vi "Test MQTT-3.1.4-2.vi"(8 "error in (no error)":errorcluster) -> (0 "error out":errorcluster)   [LabVIEW 2013]
uses:
  <vilib>/LabVIEW Open Source Project/MQTT Control Packets/Control Packets/CONNACK/Connect Return Code -- enum.ctl
  <vilib>/LabVIEW Open Source Project/MQTT Control Packets/Control Packets/CONNACK/CONNACK.lvclass
  <vilib>/LabVIEW Open Source Project/MQTT Control Packets/Control Packets/CONNECT/CONNECT.lvclass
  <vilib>/LabVIEW Open Source Project/MQTT Control Packets/Control Packets/ControlPacket/ControlPacket.lvclass
  <vilib>/addons/_JKI Toolkits/Caraya/classes/Test/Test.lvclass
  <vilib>/addons/_JKI Toolkits/Caraya/classes/Assert/Assert.lvclass
  <vilib>/LabVIEW Open Source Project/MQTT Control Packets/Control Packets/DISCONNECT/DISCONNECT.lvclass
  <vilib>/LabVIEW Open Source Project/MQTT Connection/MQTT_Connection/Connection/Connection.lvclass
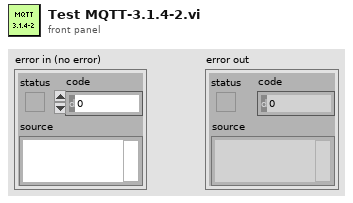
[diagram p1: front panel]
types:
  T1 = typedef "MQTT_Control_Packets.lvlib/CONNACK.lvclass/Connect Return Code -- enum.ctl" = enum16{"Connection accepted", "Unacceptable protocol version", "Identifier Rejected", "Server Unavailable", "Bad Username or Password", "Not Authorized"}
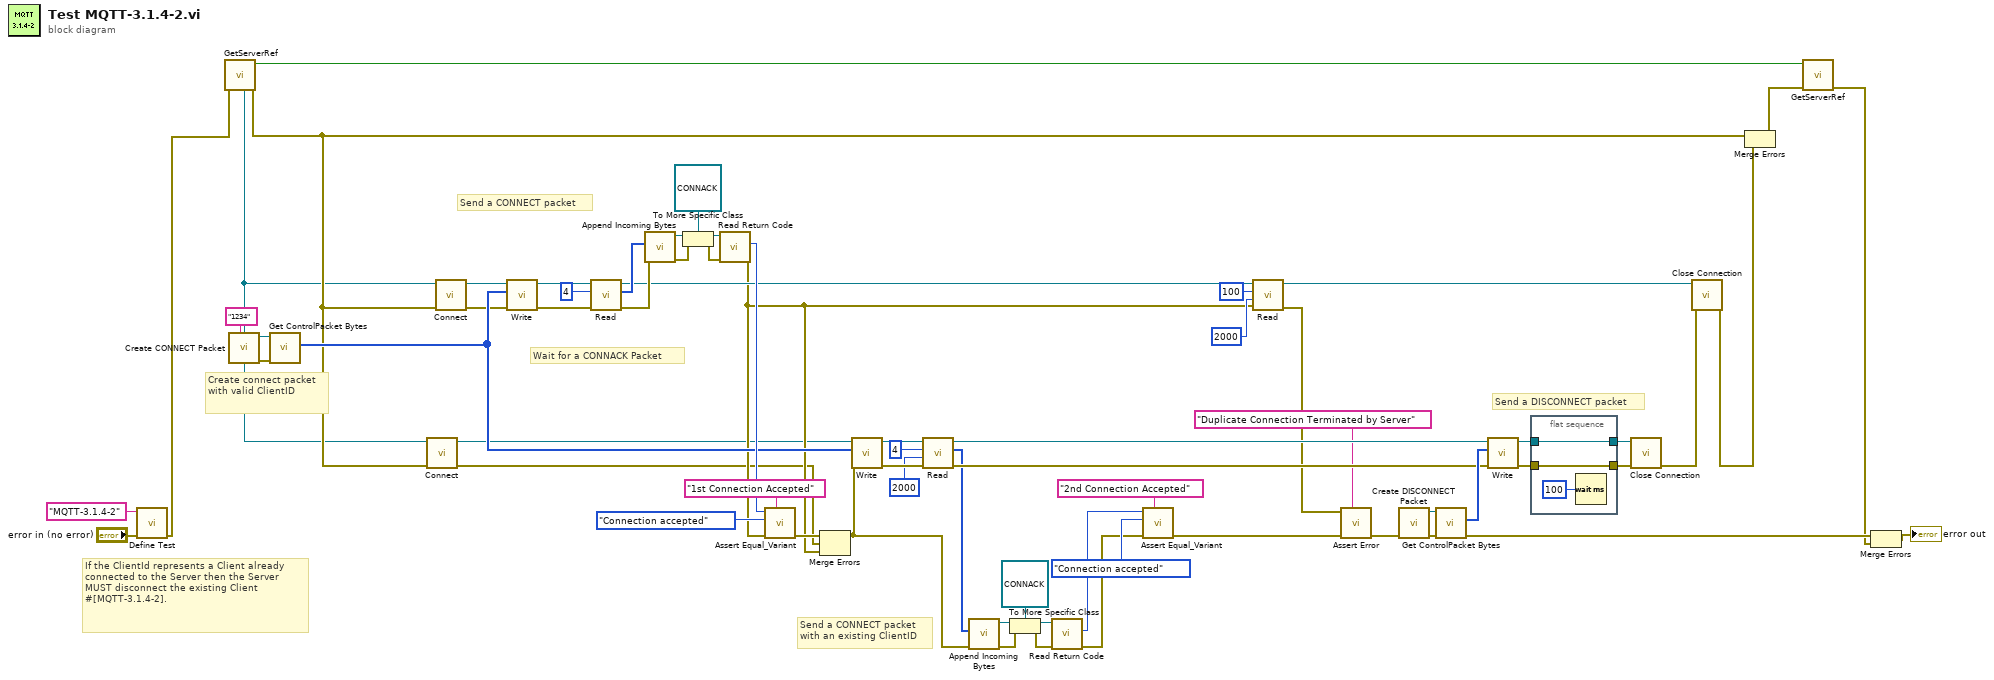
[diagram p0: block diagram]
diagram:
  # "Send a CONNECT packet\nwith an existing ClientID"
  # "If the ClientId represents a Client already connected to the Server then the Server MUST disconnect the existing Client #[MQTT-3.1.4-2]."
  # "Send a DISCONNECT packet"
  # "Wait for a CONNACK Packet"
  # "Create connect packet with valid ClientID"
  # "Send a CONNECT packet"
  n1 = call <vilib>:"Define Test.vi"("error in (no error)"="error in (no error)", "Label (VI Title)"="MQTT-3.1.4-2") -> ("error out"=w10:errorcluster)  [unwired: 9 in]
  n2 = call "GetServerRef.vi"("error in"=w10) -> ("error out"=w9:errorcluster, "Created"=w11:bool, "Connection Config"=w1:refnum<class "Connection.lvclass">)  [unwired: 6 in, 2 out]
  n3 = call <vilib>:"Create CONNECT Packet.vi"("Client ID (empty: generate new)"="1234") -> ("error out"=w66:errorcluster, "CONNECT"=w67:refnum<class "CONNECT.lvclass">)  [unwired: 8 in, 1 out]
  n4 = call <vilib>:"Get ControlPacket Bytes.vi"("error in (no error)"=w66, "ControlPacket"=w67) -> ("Bytes Stream"=w42:u8[])  [unwired: 6 in, 3 out]
  n5 = call <vilib>:"Connect.vi"("error in (no error)"=w9, "Connection in"=w1) -> ("error out"=w14:errorcluster, "Connection out"=w15:refnum<class "Connection.lvclass">)  [unwired: 8 in]
  n6 = call <vilib>:"Connect.vi"("error in (no error)"=w9, "Connection in"=w1) -> ("error out"=w12:errorcluster, "Connection out"=w13:refnum<class "Connection.lvclass">)  [unwired: 8 in]
  n7 = call <vilib>:"Write.vi"("error in (no error)"=w12, "Bytes"=w42, "Connection in"=w13) -> ("error out"=w46:errorcluster, "Connection"=w47:refnum<class "Connection.lvclass">)  [unwired: 7 in]
  n8 = call <vilib>:"Read.vi"("error in (no error)"=w46, "bytes to read (100)"=4 ("bytes to read"), "TCPConnection in"=w47) -> ("error out"=w43:errorcluster, "Bytes"=w45:u8[], "TCPConnection out"=w32:refnum<class "Connection.lvclass">)  [unwired: 4 in, 2 out]
  n9 = call <vilib>:"Append Incoming Bytes.vi"("error in (no error)"=w43, "Incoming Packets"=w45) -> ("error out"=w49:errorcluster, "ControlPacket"=w55:refnum<class "ControlPacket.lvclass">)  [unwired: 6 in, 2 out]
  n10 = To More Specific Class(target class=refnum<class "CONNACK.lvclass"> refnum ("CONNACK"), reference=w55, error in=w49) -> (specific class reference=w54:refnum<class "CONNACK.lvclass">, error out=w50:errorcluster)
  n11 = call <vilib>:"Read Return Code.vi"("error in (no error)"=w50, "CONNACK in"=w54) -> ("error out"=w16:errorcluster, "Return Code"=w52:T1)  [unwired: 7 in, 1 out]
  n12 = call <vilib>:"Assert Equal_Variant.vi"("Label"="1st Connection Accepted", "error in (no error)"=w16, "Y"=Connect_Return_Code_--_enum."Connection accepted" ("Return Code"), "X"=w52) -> ("error out"=w31:errorcluster)  [unwired: 7 in]
  n13 = Merge Errors(w31, w14, w16) -> (w19:errorcluster)
  n14 = call <vilib>:"Write.vi"("error in (no error)"=w19, "Bytes"=w42, "Connection in"=w15) -> ("error out"=w33:errorcluster, "Connection"=w40:refnum<class "Connection.lvclass">)  [unwired: 7 in]
  n15 = call <vilib>:"Read.vi"("error in (no error)"=w33, "timeout (1000 ms)"=2000, "bytes to read (100)"=4 ("bytes to read"), "TCPConnection in"=w40) -> ("error out"=w34:errorcluster, "Bytes"=w28:u8[], "TCPConnection out"=w35:refnum<class "Connection.lvclass">)  [unwired: 3 in, 2 out]
  n16 = call <vilib>:"Append Incoming Bytes.vi"("error in (no error)"=w19, "Incoming Packets"=w28) -> ("error out"=w39:errorcluster, "ControlPacket"=w36:refnum<class "ControlPacket.lvclass">)  [unwired: 6 in, 2 out]
  n17 = To More Specific Class(target class=refnum<class "CONNACK.lvclass"> refnum ("CONNACK"), reference=w36, error in=w39) -> (specific class reference=w37:refnum<class "CONNACK.lvclass">, error out=w38:errorcluster)
  n18 = call <vilib>:"Read Return Code.vi"("error in (no error)"=w38, "CONNACK in"=w37) -> ("error out"=w18:errorcluster, "Return Code"=w25:T1)  [unwired: 7 in, 1 out]
  n19 = call <vilib>:"Assert Equal_Variant.vi"("Label"="2nd Connection Accepted", "error in (no error)"=w18, "Y"=Connect_Return_Code_--_enum."Connection accepted" ("Return Code"), "X"=w25) -> ("error out"=w24:errorcluster)  [unwired: 7 in]
  n20 = call <vilib>:"Read.vi"("error in (no error)"=w16, "timeout (1000 ms)"=2000, "bytes to read (100)"=100, "TCPConnection in"=w32) -> ("error out"=w23:errorcluster, "TCPConnection out"=w6:refnum<class "Connection.lvclass">)  [unwired: 3 in, 3 out]
  n21 = call <vilib>:"Assert Error.vi"("Label"="Duplicate Connection Terminated by Server", "error in (no error)"=w24, "Error?"=w23) -> ("error out"=w21:errorcluster)  [unwired: 8 in]
  n22 = call <vilib>:"Create DISCONNECT Packet.vi"("error in (no error)"=w21) -> ("error out"=w61:errorcluster, "DISCONNECT"=w60:refnum<class "DISCONNECT.lvclass">)  [unwired: 8 in, 1 out]
  n23 = call <vilib>:"Get ControlPacket Bytes.vi"("error in (no error)"=w61, "ControlPacket"=w60) -> ("error out"=w20:errorcluster, "Bytes Stream"=w59:u8[])  [unwired: 6 in, 2 out]
  n24 = call <vilib>:"Write.vi"("error in (no error)"=w34, "Bytes"=w59, "Connection in"=w35) -> ("error out"=w57:errorcluster, "Connection"=w58:refnum<class "Connection.lvclass">)  [unwired: 7 in]
  n25 = flat-sequence {
    tunnel: w58 -> [w70]
    tunnel: [w70] -> w56
    tunnel: [w68] -> w53
    tunnel: w57 -> [w68]
    frame #0 {
      n26 = Wait (ms)(milliseconds to wait=u32 100) -> ()  [unwired: 1 out]
    }
  }
  n27 = call <vilib>:"Close Connection.vi"("error in (no error)"=w53, "Connection in"=w56) -> ("error out"=w5:errorcluster)  [unwired: 8 in, 1 out]
  n28 = call <vilib>:"Close Connection.vi"("error in (no error)"=w5, "Connection in"=w6) -> ("error out"=w4:errorcluster)  [unwired: 8 in, 1 out]
  n29 = Merge Errors(w9, w4) -> (w8:errorcluster)
  n30 = call "GetServerRef.vi"("error in"=w8, "Destroy (F)"=w11) -> ("error out"=w7:errorcluster)  [unwired: 5 in, 4 out]
  n31 = Merge Errors(w20, w7) -> (→"error out":errorcluster)
